vi "myRIO_BRig_Host_endExp_filePath__storeLocation.vi"(9 "input_expPrefix":string, 10 "input_fileName":string, 11 "input_filePath_storage":string) -> (1 "output_filePath":string)   [LabVIEW 2014]
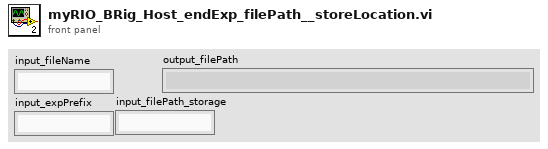
[diagram p1: front panel]
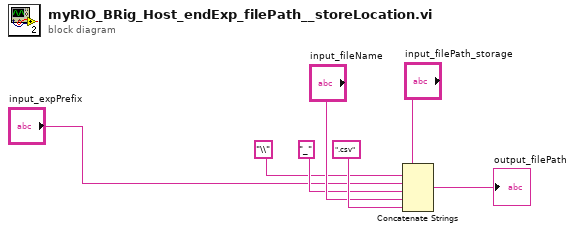
[diagram p0: block diagram]
diagram:
  n1 = Concatenate Strings("input_filePath_storage", "\\" ("string"), "input_expPrefix", "_" ("string"), "input_fileName", ".csv" ("string")) -> (→"output_filePath":string)
